vi "Change Camera.vi"(8 "error in (no error)":errorcluster, 10 "New Camera":string, 11 "HIJ Vision Camera App In":refnum<class "HIJ Vision Camera App.lvclass">) -> (0 "error out":errorcluster, 3 "HIJ Vision Camera App Out":refnum<class "HIJ Vision Camera App.lvclass">)   [LabVIEW 2014, in "HIJ Vision Camera App.lvlib" / "HIJ Vision Camera App.lvclass"]
uses:
  HIJ Vision Camera App.lvclass
  HIJ Vision Camera App.lvclass/HIJ Vision Camera App.ctl
  HIJ Vision Application/HIJ Vision Application/HIJ Vision Application.lvclass/HIJ Vision Application.ctl
  Camera Actors/Camera Actor/Camera Actor Messages/Change Camera Msg/Change Camera Msg.lvclass/Change Camera Msg.ctl
  <vilib>/ActorFramework/Message Enqueuer/Message Enqueuer.lvclass/Message Enqueuer.ctl
  Display Actors/HIJ Vision Display/HIJ Vision Display Messages/Change Image Source Msg/Change Image Source Msg.lvclass/Change Image Source Msg.ctl
  HIJ Vision Application/HIJ Vision Application/Read Display Enq.vi
  <vilib>/ActorFramework/Message Enqueuer/Enqueue.vi
  <vilib>/ActorFramework/Message Priority Queue/Priority Enqueue.vi
  <vilib>/ActorFramework/Message Enqueuer/Message Enqueuer.lvclass
  Camera Actors/Camera Actor/Camera Actor Messages/Change Camera Msg/Change Camera Msg.lvclass
  Display Actors/HIJ Vision Display/HIJ Vision Display Messages/Change Image Source Msg/Change Image Source Msg.lvclass
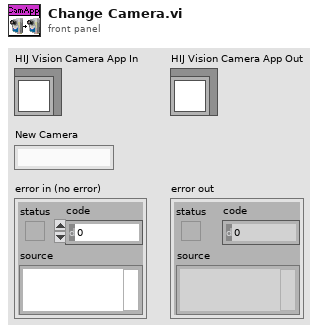
[diagram p1: front panel]
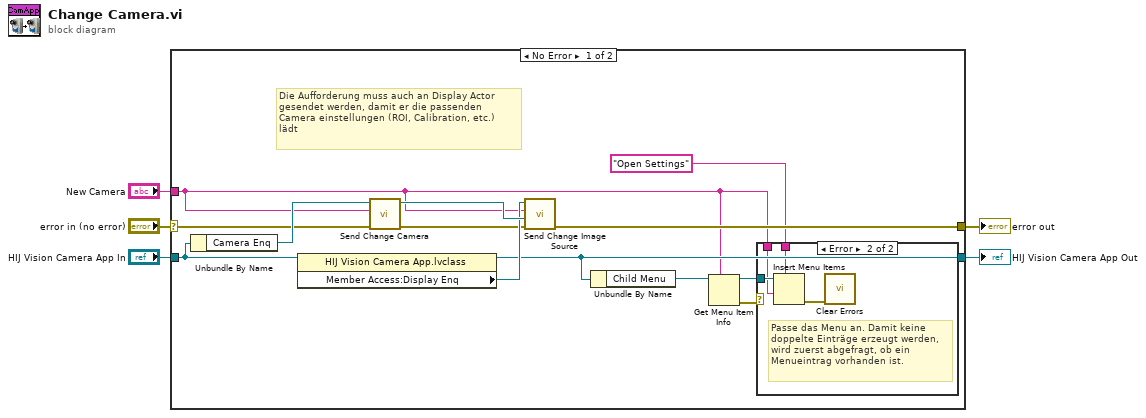
[diagram p0: block diagram]
diagram:
  n1 = case shown="No Error" "error in (no error)" {
    selector: "error in (no error)" -> [w13 w24]
    tunnel: [w12 w24] -> w4
    tunnel: [w11 w23] -> w2
    tunnel: "HIJ Vision Camera App In" -> [w17 w23]
    tunnel: "New Camera" -> [w7 _]
    frame No Error {
      # "Die Aufforderung muss auch an Display Actor\ngesendet werden, damit er die passenden \nCamera einstellungen (ROI, Calibration, etc.)\nlädt"
      n2 = Unbundle By Name(w17) -> ("Camera Enq"=w16:refnum<class "Message Enqueuer.lvclass">)
      n3 = property class="HIJ Vision Camera App.lvclass"(reference=w17) -> (reference out=w11:refnum<class "HIJ Vision Camera App.lvclass">, "Member Access:Display Enq"=w15:refnum<class "Message Enqueuer.lvclass">)  [unwired: 1 in, 1 out]
      n4 = call "Send Change Camera.vi"("error in (no error)"=w13, "New Camera"=w7, "Message Enqueuer"=w16) -> ("error out"=w14:errorcluster, "Message Enqueuer out"=w18:refnum<class "Message Enqueuer.lvclass">)  [unwired: 7 in]
      n5 = call "Send Change Image Source.vi"("error in (no error)"=w14, "Image Source Enq"=w18, "Image Source"=w7, "Message Enqueuer"=w15) -> ("error out"=w12:errorcluster)  [unwired: 6 in, 1 out]
      n6 = Unbundle By Name(w11) -> ("Child Menu"=w10:refnum<k9>)
      n7 = Get Menu Item Info(7:w7, 11:w10) -> (0:w6:errorcluster, 3:w8:refnum<k9>)  [unwired: 1 in, 5 out]
      n8 = case shown="Error" w6 {
        tunnel: "Open Settings" ("menu tag") -> [_ w22]
        tunnel: w8 -> [_ w20]
        tunnel: w7 -> [_ w19]
        frame No Error {
        }
        frame Error {
          # "Passe das Menu an. Damit keine \ndoppelte Einträge erzeugt werden,\nwird zuerst abgefragt, ob ein \nMenueintrag vorhanden ist."
          n9 = Insert Menu Items(5:w22, 7:w19, 9:w20) -> (0:w21:errorcluster)  [unwired: 3 in, 2 out]
          n10 = call <vilib>:"Clear Errors.vi"("error in (no error)"=w21) -> ()  [unwired: 5 in, 2 out]
        }
      }
    }
    frame Error {
    }
  }
  "error out" <- w4
  "HIJ Vision Camera App Out" <- w2
